vi "init lvdt comms.vi"(7 "rs232?":bool, 8 "error in":errorcluster, 10 "LVDT Unit 1 ip":string, 11 "VISA Refnum in":refnum<visa-resource-name>) -> (0 "error out":errorcluster, 3 "VISA resource name out":refnum<visa-resource-name>)   [LabVIEW 2018]
uses:
  <vilib>/Instr/_visa.llb/VISA Configure Serial Port (Instr).vi
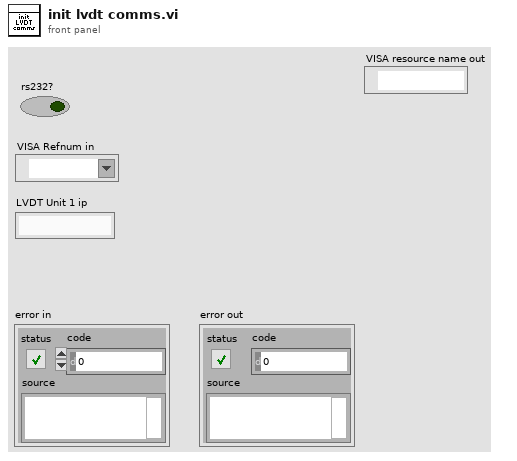
[diagram p1: front panel]
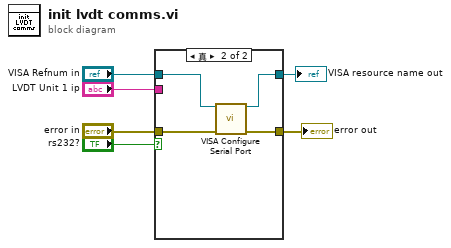
[diagram p0: block diagram]
diagram:
  n1 = case shown="真" "rs232?" {
    tunnel: "error in" -> [w7 w11]
    tunnel: [w7 w10] -> w4
    tunnel: "LVDT Unit 1 ip" -> [_ _]
    tunnel: "VISA Refnum in" -> [w8 w12]
    tunnel: [w8 w9] -> w1
    frame False {
    }
    frame True {
      n2 = call-poly "VISA Configure Serial Port"("VISA resource name"=w12, "error in (no error)"=w11) -> ("VISA resource name out"=w9:refnum<visa-resource-name>, "error out"=w10:errorcluster)  [unwired: 12 in]
    }
  }
  "error out" <- w4
  "VISA resource name out" <- w1
